vi "KE Timer -- Simple Timer tmp.vi"(0 "Resource In":refnum<visa-resource-name>, 2 "TIn (ms)":u32, 5 "error in (no error)":errorcluster, 8 "Action":enum16{"Set TStart to TCurrent", "Get Deltas"}(ring)) -> (7 "TStart (s)":dbl, 9 "TCurrent (s)":dbl, 11 "TCurrent - TStart (s)":dbl, 13 "TCurrent - TIn (s)":dbl, 14 "Resource Out (dupl)":refnum<visa-resource-name>, 15 "TStart (ms)":u32, 16 "TCurrent (ms)":u32, 17 "TCurrent - TStart (ms)":u32, 18 "TCurrent - TIn (ms)":u32, 19 "error out (dupl)":errorcluster)   [LabVIEW 2014, in "Keithley 622x tmp.lvlib"]
doc: "Implements a simple timer."
uses:
  Keithley 622x tmp.lvlib
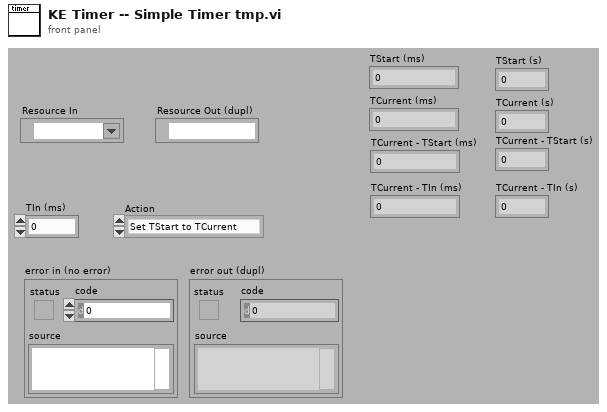
[diagram p1: front panel]
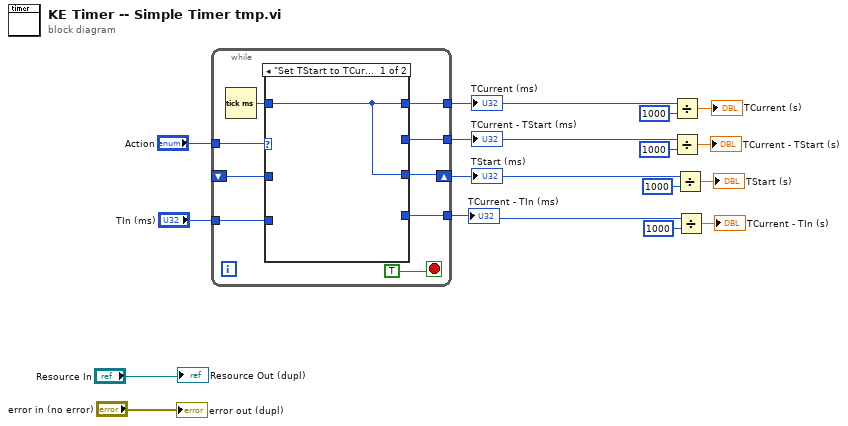
[diagram p0: block diagram]
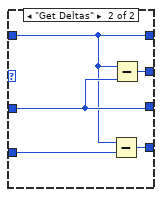
[diagram p2: hidden frame]
diagram:
  n1 = while {
    shift-right: [w24] -> w7
    shift-left: _ -> [w23]
    tunnel: "Action" -> [w25]
    tunnel: [w22] -> w15
    tunnel: "TIn (ms)" -> [w20]
    tunnel: [w19] -> w4
    tunnel: [w18] -> w2
    stop <- TRUE stop-if-true
    n2 = Tick Count (ms)() -> (millisecond timer value=w17:u32)
    n3 = case shown="\"Set TStart to TCurrent\"" w25 {
      tunnel: [w26 w30] -> w24
      tunnel: w23 -> [_ w30]
      tunnel: [_ w31] -> w22
      tunnel: w20 -> [_ w29]
      tunnel: [_ w28] -> w19
      tunnel: [w26 w27] -> w18
      tunnel: w17 -> [w26 w27]
      frame "Set TStart to TCurrent" {
      }
      frame "Get Deltas" {
        n4 = Subtract(x=w27, y=w29) -> (x-y=w28:u32)
        n5 = Subtract(x=w27, y=w30) -> (x-y=w31:u32)
      }
    }
  }
  "TStart (ms)" <- w7
  "TCurrent - TStart (ms)" <- w15
  "TCurrent - TIn (ms)" <- w4
  "TCurrent (ms)" <- w2
  n6 = Divide(x=w2, y=u32 1000) -> (x/y=→"TCurrent (s)":dbl)
  n7 = Divide(x=w15, y=u32 1000) -> (x/y=→"TCurrent - TStart (s)":dbl)
  n8 = Divide(x=w7, y=u32 1000) -> (x/y=→"TStart (s)":dbl)
  n9 = Divide(x=w4, y=u32 1000) -> (x/y=→"TCurrent - TIn (s)":dbl)
  "error out (dupl)" <- "error in (no error)"
  "Resource Out (dupl)" <- "Resource In"
